vi "Create.vi"(7 "Minimum Number of Calls":u32, 8 "error in (no error)":errorcluster, 10 "Comparator":refnum<class "Comparator.lvclass">) -> (0 "error out":errorcluster, 3 "At Least Out":refnum<class "At Least.lvclass">)   [LabVIEW 2020, in "At Least.lvlib" / "At Least.lvclass"]
uses:
  At Least.lvclass
  Core/Comparator/Comparator.lvclass
  At Least.lvclass/At Least.ctl
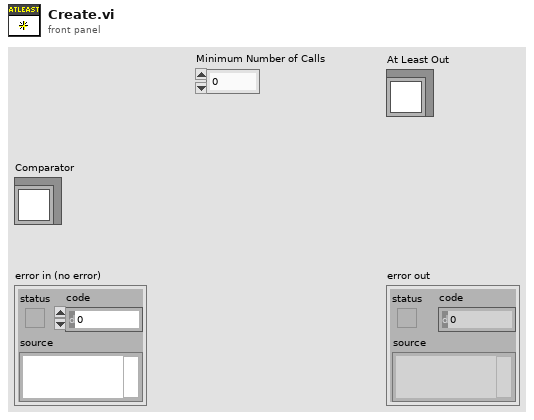
[diagram p1: front panel]
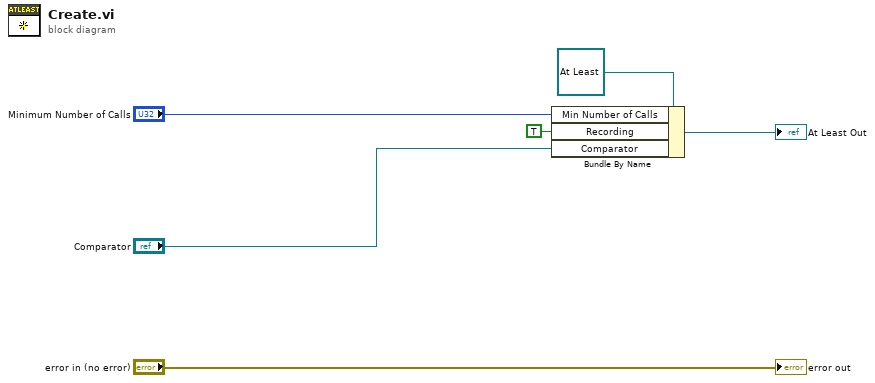
[diagram p0: block diagram]
diagram:
  n1 = Bundle By Name(cluster=refnum<class "At Least.lvclass"> refnum ("One or More"), "Min Number of Calls"="Minimum Number of Calls", "Recording"=TRUE, "Comparator"="Comparator") -> (→"At Least Out":refnum<class "At Least.lvclass">)
  "error out" <- "error in (no error)"
